vi "Profile Editor_Beta1 - Drag-n-Drop - Custom Data.vi"() -> ()   [LabVIEW 2010]
doc: "This VI illustrates the use of a built-in Drag and Drop source with custom Drag and Drop data and a custom target. \n\nThe various events that are triggered are listed here:\n\n------------------\nDrag Starting?\n------------------\n\nThe \"Drag Starting?\" event is triggered when a drag begins. This is a source-side event.\n\nDrag Data is passed as an array of 2-element clusters containing a \"drag name\" and variant\n\"drag data.\"\n\n\n-------------\nDrag Enter\n-------------\n\nThe \"Drag Enter\" event is triggered when a Drag and Drop enters any control or indicator. This is a target-side event.\n\nThe Available Data Names are searched for a name that matches the expected data name.\n\nIf a match is found the Drag enter is accepted and the cursor is changed to indicate that a valid drop target has been found.\n\n\n------\nDrop\n------\n\nThe \"Drop\" event is triggered when a Drag and Drop ends within a control or indicator. This is a target-side event.\n\nA Drag and Drop \"data name\" and \"data type\" prototype are given to extract the original data from the array and convert from variant to the intended data type.\n\nThe Get Drag Drop Data VI is used for this process."
uses:
  <vilib>/Utility/miscctls.llb/LVPoint32TypeDef.ctl
  <vilib>/Analysis/NI_AALBase.lvlib
panel:
  out "Coords":T1
  out "XY Current":cluster{"X":dbl, "Y":dbl}
  out "Formatted Parameters String":string
  in  "Tab Control":T2(tab)
  in  "Sine":T3={"samples"=128, "amplitude"=1.0, "frequency"=0.0078125, "phase in"=0.0, "reset phase"=TRUE} {"phase in" format="%0.2f"; "frequency" format="%0.4e"; "amplitude" format="%0.2f"}
  in  "Square":T4={"samples"=128, "amplitude"=1.0, "frequency"=0.0078125, "phase in"=0.0, "reset phase"=TRUE, "duty cycle (%)"=50.0} {"duty cycle (%)" format="%0.2f"; "phase in" format="%0.2f"; "frequency" format="%0.4e"; "amplitude" format="%0.2f"}
  in  "Sawtooth":T3={"samples"=128, "amplitude"=1.0, "frequency"=0.0078125, "phase in"=0.0, "reset phase"=TRUE} {"phase in" format="%0.2f"; "frequency" format="%0.4e"; "amplitude" format="%0.2f"}
  in  "Triangle":T3={"samples"=128, "amplitude"=1.0, "frequency"=0.0078125, "phase in"=0.0, "reset phase"=TRUE} {"phase in" format="%0.2f"; "frequency" format="%0.4e"; "amplitude" format="%0.2f"}
  in  "Sequence Table":string[][](table)
  in  "parameter description":string="This area, is either for a cluster,\nor tab of clusters, or possibly a\nSubPanel, to allow entry / edit of\nthe parameters of a Step.\n\nEX: RAMP\n      Start Type: Current Value\n                         Abs Value\n      Rate:  Deg/Unit Time\n      End Type:   Time, Target Val\n\nEX: HOLD\n      Type:  Duration Time or \n                 Clock Time or\n                 Variable Trigger\n      Time:  Duration\n      Time:  Clock Date:Hr:Min:Sec\n      Trigger:  VarName, Val, <=>"
  out "XY Dropped":cluster{"X":dbl, "Y":dbl}
  in  "message":string="Drop not Allowed"
  in  "stop":bool
  out "Waveform Chart":dbl[](graph)
  in  "Signals":string(tree)
  # "This VI illustrates the use of a built-in Drag and Drop source with custom Drag and Drop data.  \nThe signal names in the Tree control are draggable items that will produce their corresponding \nsignals when dropped on the Waveform Chart indicator.\n\nInstructions:\n1) Run the VI\n2) Drag The signals (i.e. Sine) from the tree control to the Waveform Chart\n3) Stop the VI and look at the Block Diagram for more information"
  # "Buttons for New, Open, Save\nMacroName, Run, Pause, Stop\nHelp?"
  # "Step Parameters"
  # "Instead of Sine, Square, etc, we would have the step types for and Ramp-n-Soak profile:\nStart, Stop, RampUp, RampDown, Hold_Time, Hold_Trigger,\n\nControl Steps: Repeat [FOR | WHILE | UNTIL]\n\nMake generalizable.\n\nWhen you select a Step Type, the appropriate variables cluster shows up in the Parameters\nbox, to the right of the Tree, you change the parameters, then drag either to the Step Table,\nor to the Waveform, to insert into the sequence.\n\nIf you click on the table/list, or the Chart, then the selected item segment type is looked up,\nand that is what the Tree and Parameters cluster is set too.\n\nAdd:  Save/Restore."
  # "May want to use a MCLB instead\nof a table. May not want the\ntable to be directly editable, but\nonly through the Tree/Param ??"
  # "This is the default. Select one of\nthe Signal Types in the Tree to the\nleft, then fill in the parameters in\nthe cluster here, before dragging to\nthe Waveform Chart or the \nSequence Table"
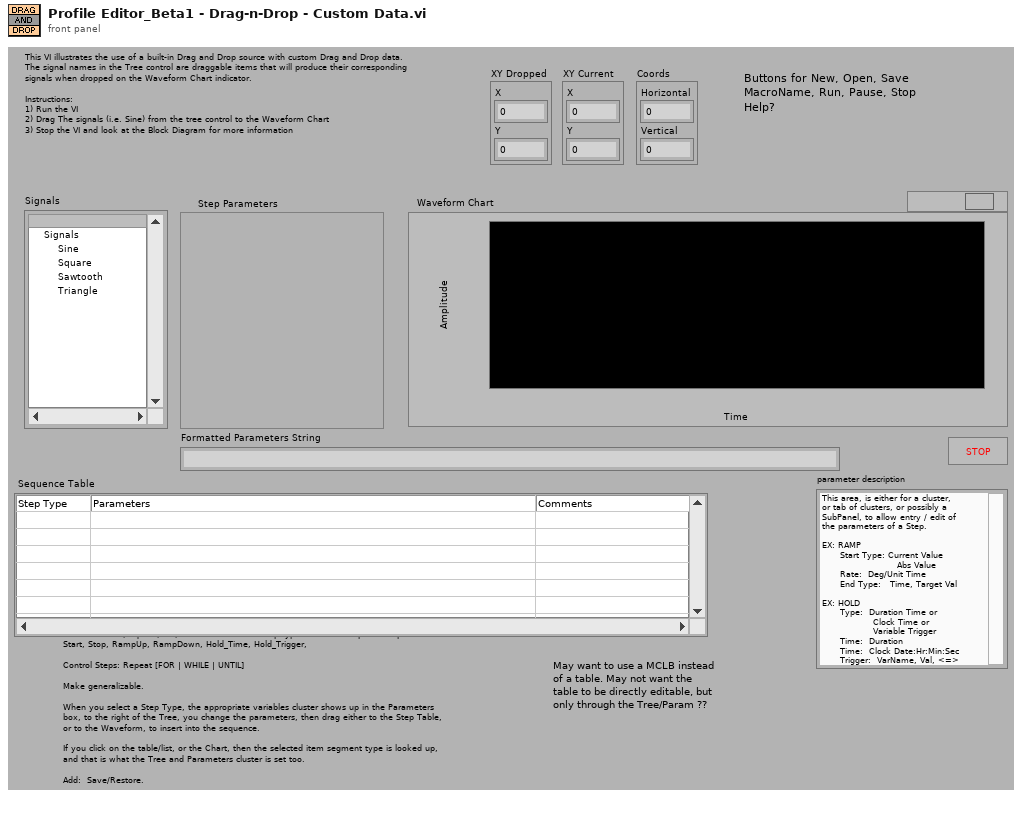
[diagram p1: front panel]
types:
  T1 = typedef "LVPoint32TypeDef.ctl" = cluster{"Horizontal":i32, "Vertical":i32}
  T2 = enum32{"Signals", "Sine", "Square", "Sawtooth", "Triangle"}
  T3 = cluster{"samples":i32, "amplitude":dbl, "frequency":dbl, "phase in":dbl, "reset phase":bool}
  T4 = cluster{"samples":i32, "amplitude":dbl, "frequency":dbl, "phase in":dbl, "reset phase":bool, "duty cycle (%)":dbl}
  T5 = cluster{"data name":string, "drag data":variant}[]
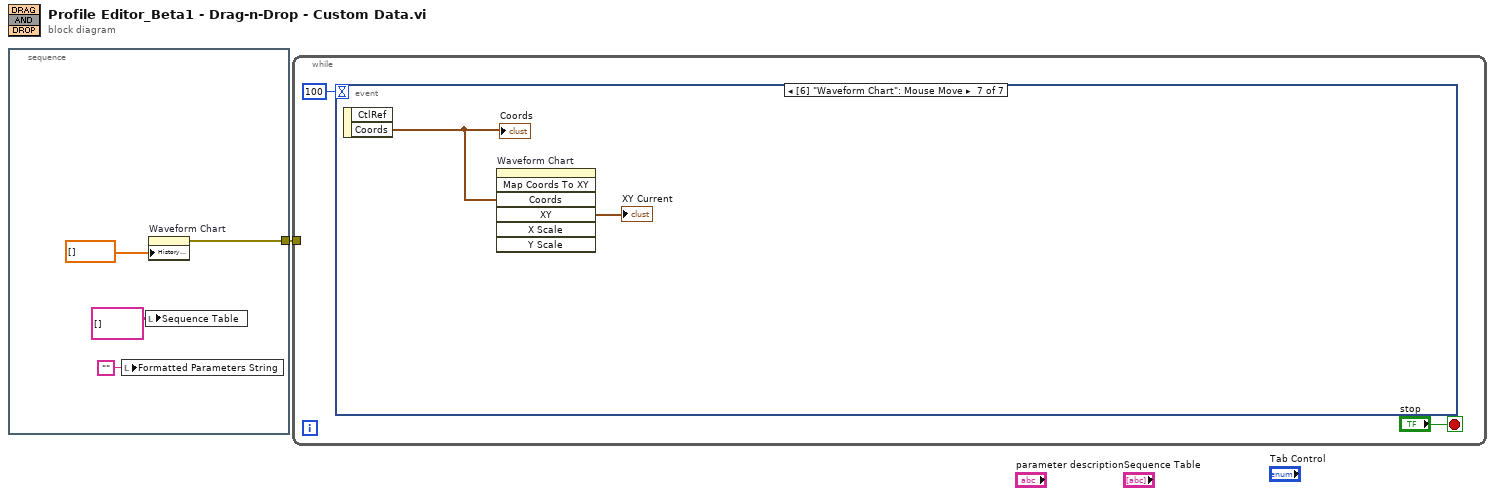
[diagram p0: block diagram]
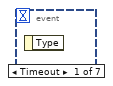
[diagram p2: hidden frame]
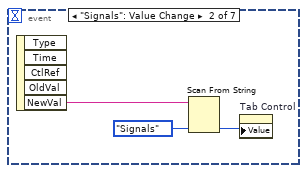
[diagram p3: hidden frame]
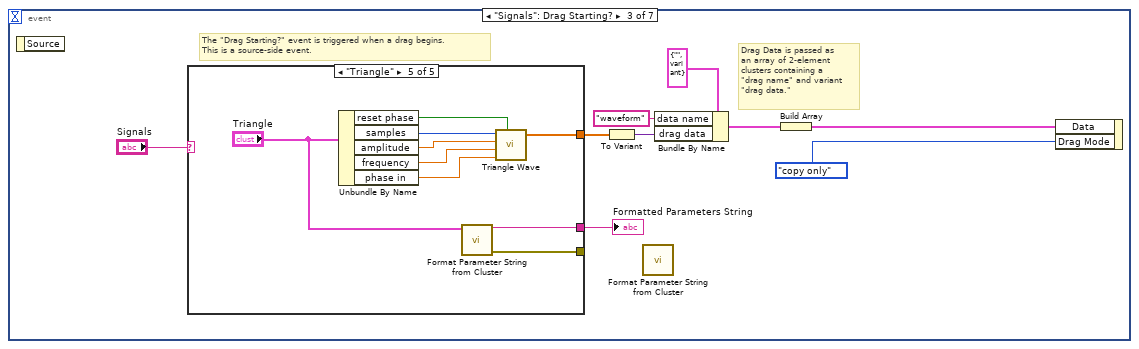
[diagram p4: hidden frame]
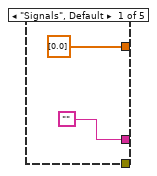
[diagram p5: hidden frame]
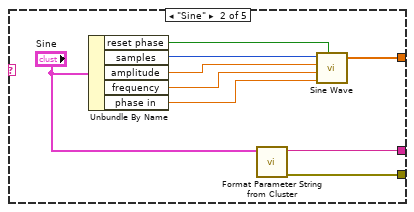
[diagram p6: hidden frame]
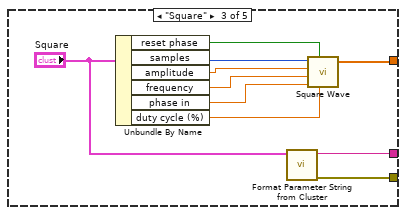
[diagram p7: hidden frame]
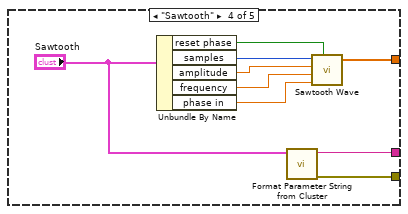
[diagram p8: hidden frame]
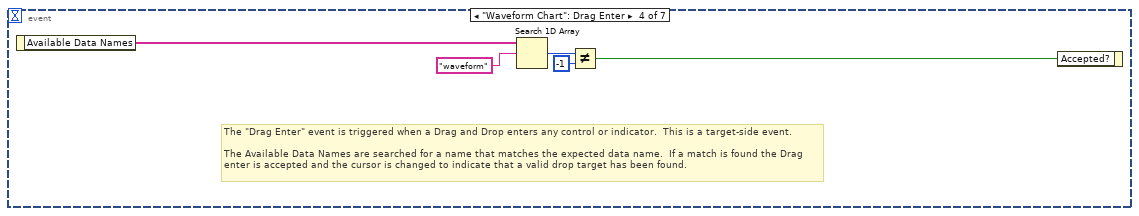
[diagram p9: hidden frame]
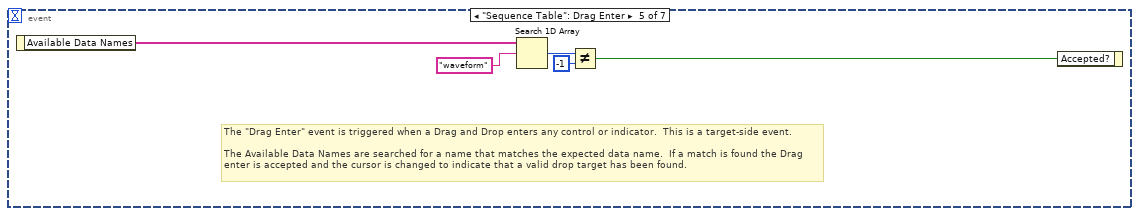
[diagram p10: hidden frame]
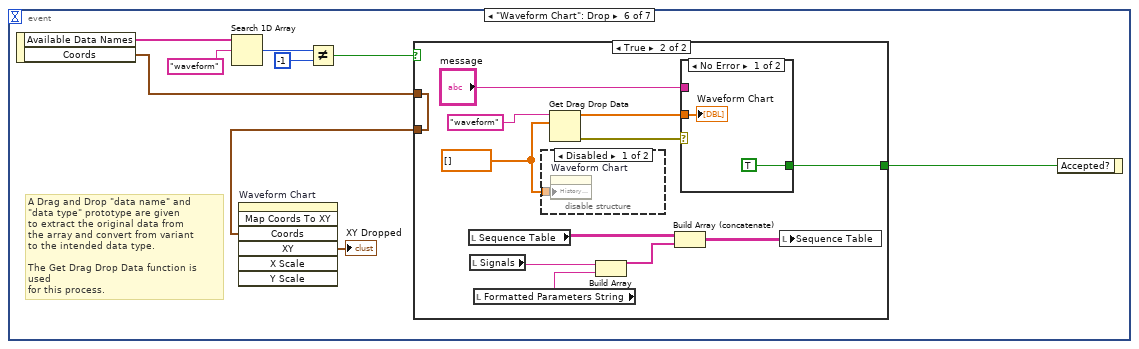
[diagram p11: hidden frame]
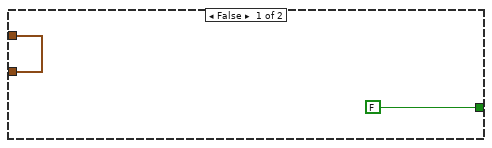
[diagram p12: hidden frame]
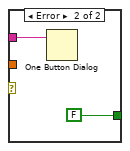
[diagram p14: hidden frame]
diagram:
  n1 = stacked-sequence {
    tunnel: [w4] -> w1
    frame #0 {
      n2 = local write "Formatted Parameters String"("") -> ()
      n3 = local write "Sequence Table"(string[][] [] ("Sequence Table")) -> ()
      n4 = property on="Waveform Chart" class="WFChart (strict)"("History Data"=dbl[] []) -> (error out=w4:errorcluster)  [unwired: 2 in, 1 out]
    }
  }
  n5 = while {
    tunnel: w1 -> [_]
    stop <- "stop" stop-if-true
    n6 = event shown="[6] \"Waveform Chart\": Mouse Move" {
      selector: _ -> [_ _ _ _ _ _ _]
      dyn-events: _ -> [_ _ _ _ _ _ _]
      timeout: 100 -> [_ _ _ _ _ _ _]
      event Timeout {
        n7 = event-data() -> ()  [unwired: 1 in, 1 out]
      }
      event "Signals": Value Change {
        n8 = event-data() -> ("NewVal"=w10:string)  [unwired: 1 in, 4 out]
        n9 = Scan From String(input string=w10, default 1=T2."Signals" ("Tab Control")) -> (output 1=w8:T2)  [unwired: 3 in, 3 out]
        n10 = property on="Tab Control" class="TabCtl (strict)"("Value"=w8) -> ()  [unwired: 2 in, 2 out]
      }
      event "Signals": Drag Starting? {
        # "Drag Data is passed as\nan array of 2-element\nclusters containing a \n\"drag name\" and variant\n\"drag data.\""
        # "The \"Drag Starting?\" event is triggered when a drag begins.\nThis is a source-side event."
        n11 = event-data() -> ()  [unwired: 1 in, 1 out]
        n12 = case shown="\"Triangle\"" "Signals" {
          tunnel: [dbl[] [0.0] w30 w40 w49 w58] -> w16
          tunnel: ["" w24 w32 w42 w51] -> w11
          tunnel: [_ w23 w33 w43 w50] -> _
          frame "Signals", Default {
          }
          frame "Sine" {
            n13 = Unbundle By Name("Sine") -> ("reset phase"=w28:bool, "samples"=w29:i32, "amplitude"=w27:dbl, "frequency"=w26:dbl, "phase in"=w25:dbl)
            n14 = call "Format Parameter String from Cluster.vi"("Variant"="Sine") -> ("error out"=w23:errorcluster, "String"=w24:string)  [unwired: 9 in]
            n15 = call <vilib>:"Sine Wave.vi"("samples"=w29, "amplitude"=w27, "frequency"=w26, "phase in"=w25, "reset phase"=w28) -> ("sine wave"=w30:dbl[])  [unwired: 2 out]
          }
          frame "Square" {
            n16 = Unbundle By Name("Square") -> ("reset phase"=w39:bool, "samples"=w38:i32, "amplitude"=w37:dbl, "frequency"=w36:dbl, "phase in"=w35:dbl, "duty cycle (%)"=w34:dbl)
            n17 = call "Format Parameter String from Cluster.vi"("Variant"="Square") -> ("error out"=w33:errorcluster, "String"=w32:string)  [unwired: 9 in]
            n18 = call <vilib>:"Square Wave.vi"("samples"=w38, "reset phase"=w39, "amplitude"=w37, "frequency"=w36, "duty cycle (%)"=w34, "phase in"=w35) -> ("square wave"=w40:dbl[])  [unwired: 2 out]
          }
          frame "Sawtooth" {
            n19 = Unbundle By Name("Sawtooth") -> ("reset phase"=w48:bool, "samples"=w47:i32, "amplitude"=w46:dbl, "frequency"=w45:dbl, "phase in"=w44:dbl)
            n20 = call "Format Parameter String from Cluster.vi"("Variant"="Sawtooth") -> ("error out"=w43:errorcluster, "String"=w42:string)  [unwired: 9 in]
            n21 = call <vilib>:"Sawtooth Wave.vi"("samples"=w47, "amplitude"=w46, "frequency"=w45, "phase in"=w44, "reset phase"=w48) -> ("sawtooth wave"=w49:dbl[])  [unwired: 2 out]
          }
          frame "Triangle" {
            n22 = Unbundle By Name("Triangle") -> ("reset phase"=w56:bool, "samples"=w57:i32, "amplitude"=w55:dbl, "frequency"=w54:dbl, "phase in"=w53:dbl)
            n23 = call "Format Parameter String from Cluster.vi"("Variant"="Triangle") -> ("error out"=w50:errorcluster, "String"=w51:string)  [unwired: 9 in]
            n24 = call <vilib>:"Triangle Wave.vi"("samples"=w57, "amplitude"=w55, "frequency"=w54, "phase in"=w53, "reset phase"=w56) -> ("triangle wave"=w58:dbl[])  [unwired: 2 out]
          }
        }
        "Formatted Parameters String" <- w11
        n25 = To Variant(anything=w16) -> (Variant=w17:variant)
        n26 = call "Format Parameter String from Cluster.vi"() -> ()  [unwired: 10 in, 2 out]
        n27 = Bundle By Name(cluster=cluster{"data name":string, "drag data":variant} {"data name"="", "drag data"=variant}, "data name"="waveform", "drag data"=w17) -> (w14:cluster{"data name":string, "drag data":variant})
        n28 = Build Array(w14) -> (w13:T5)
        n29 = event-data("Data"=w13, "Drag Mode"=enum32{"copy or move", "copy only", "move only"}."copy only" ("DragMode")) -> ()  [unwired: 1 in, 1 out]
      }
      event "Waveform Chart": Drag Enter {
        # "The \"Drag Enter\" event is triggered when a Drag and Drop enters any control or indicator.  This is a target-side event.\n\nThe Available Data Names are searched for a name that matches the expected data name.  If a match is found the Drag enter is accepted and the cursor is changed to indicate that a valid drop target has been found."
        n30 = event-data() -> ("Available Data Names"=w63:string[])  [unwired: 1 in]
        n31 = Search 1D Array(1D array=w63, element="waveform") -> (index of element=w61:i32)  [unwired: 1 in]
        n32 = Not Equal?(x=w61, y=-1) -> (x != y?=w59:bool)
        n33 = event-data("Accepted?"=w59) -> ()  [unwired: 1 in, 1 out]
      }
      event "Sequence Table": Drag Enter {
        # "The \"Drag Enter\" event is triggered when a Drag and Drop enters any control or indicator.  This is a target-side event.\n\nThe Available Data Names are searched for a name that matches the expected data name.  If a match is found the Drag enter is accepted and the cursor is changed to indicate that a valid drop target has been found."
        n34 = event-data() -> ("Available Data Names"=w68:string[])  [unwired: 1 in]
        n35 = Search 1D Array(1D array=w68, element="waveform") -> (index of element=w66:i32)  [unwired: 1 in]
        n36 = Not Equal?(x=w66, y=-1) -> (x != y?=w64:bool)
        n37 = event-data("Accepted?"=w64) -> ()  [unwired: 1 in, 1 out]
      }
      event "Waveform Chart": Drop {
        # "A Drag and Drop \"data name\" and \n\"data type\" prototype are given\nto extract the original data from \nthe array and convert from variant\nto the intended data type.\n\nThe Get Drag Drop Data function is used\nfor this process."
        n38 = event-data() -> ("Available Data Names"=w77:string[], "Coords"=w70:T1)  [unwired: 1 in]
        n39 = Search 1D Array(1D array=w77, element="waveform") -> (index of element=w75:i32)  [unwired: 1 in]
        n40 = Not Equal?(x=w75, y=-1) -> (x != y?=w73:bool)
        n41 = case shown="True" w73 {
          tunnel: [FALSE w86] -> w72
          tunnel: w70 -> [w78 w85]
          tunnel: [w78 w85] -> w69
          frame False {
          }
          frame True {
            w91 = dbl[] []
            n42 = local read "Sequence Table"() -> (w84:string[][])
            n43 = local read "Signals"() -> (w82:string)
            n44 = local read "Formatted Parameters String"() -> (w80:string)
            n45 = disable-structure shown="Disabled" {
              disable-tunnel: w91 -> [w92 _]
              frame Disabled {
                n46 = property on="Waveform Chart" class="WFChart (strict)"("History Data"=w92) -> ()  [unwired: 2 in, 2 out]
              }
              frame Enabled {
              }
            }
            n47 = Get Drag Drop Data(8:w91, 9:"waveform" ("data name")) -> (0:w88:errorcluster, 3:w89:dbl[])  [unwired: 1 in]
            n48 = Build Array(w82, w80) -> (w81:string[])
            n49 = Build Array (concatenate)(w84, w81) -> (w83:string[][])
            n50 = case shown="No Error" w88 {
              tunnel: w89 -> [w93 _]
              tunnel: [TRUE FALSE] -> w86
              tunnel: "message" -> [_ w95]
              frame No Error {
                "Waveform Chart" <- w93
              }
              frame Error {
                n51 = One Button Dialog(message=w95) -> ()  [unwired: 1 in, 1 out]
              }
            }
            n52 = local write "Sequence Table"(w83) -> ()
          }
        }
        n53 = invoke on="Waveform Chart" class="WFChart (strict)" method="Map Coords To XY"("Coords"=w69) -> ("XY"=→"XY Dropped":cluster{"X":dbl, "Y":dbl})  [unwired: 6 in, 6 out]
        n54 = event-data("Accepted?"=w72) -> ()  [unwired: 1 in, 1 out]
      }
      event "Waveform Chart": Mouse Move {
        n55 = event-data() -> ("Coords"=w98:T1)  [unwired: 1 in, 1 out]
        "Coords" <- w98
        n56 = invoke on="Waveform Chart" class="WFChart (strict)" method="Map Coords To XY"("Coords"=w98) -> ("XY"=→"XY Current":cluster{"X":dbl, "Y":dbl})  [unwired: 6 in, 6 out]
      }
    }
  }
